vi "PDP Currents Variable.vi"() -> ()   [LabVIEW 2016]
panel:
  out "Array":dbl[](array[numeric])
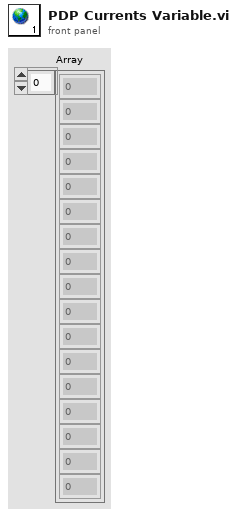
[diagram p1: front panel]
diagram:
